vi "Queue Remove.vi"(6 "timeout(ms: -1)":i32=-1, 8 "error in (no error)":errorcluster, 11 "queue name":string) -> (0 "error out":errorcluster, 1 "timeout？":bool, 2 "data":variant, 3 "event":string)   [LabVIEW 2020]
uses:
  Control/Queue Data.ctl
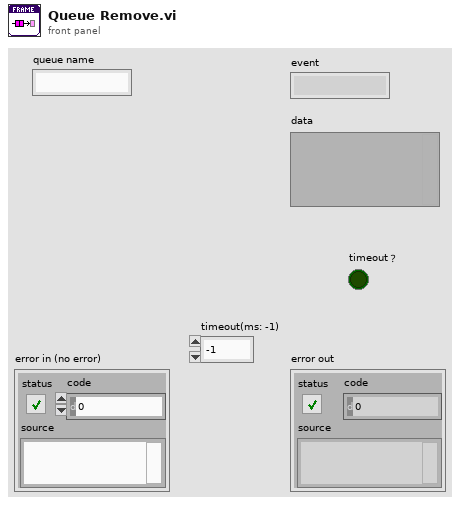
[diagram p1: front panel]
types:
  T1 = typedef "Queue Data.ctl" = cluster{"event":string, "data":variant}
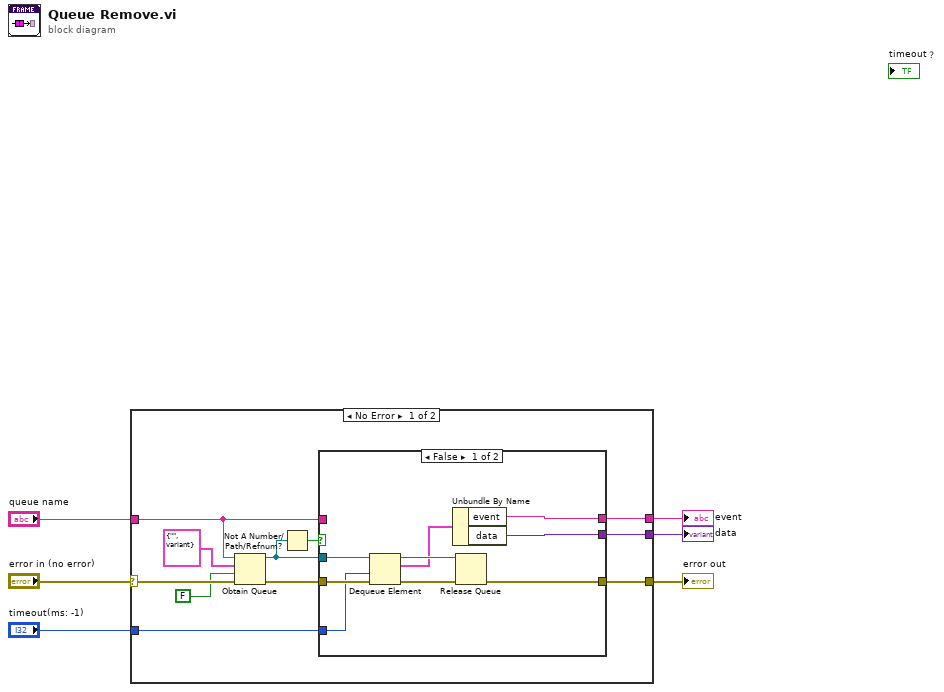
[diagram p0: block diagram]
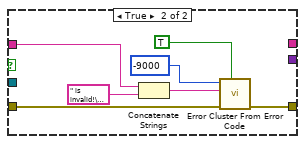
[diagram p2: hidden frame]
diagram:
  n1 = case shown="No Error" "error in (no error)" {
    selector: "error in (no error)" -> [w17 w34]
    tunnel: [w11 w34] -> w5
    tunnel: "queue name" -> [w12 _]
    tunnel: "timeout(ms: -1)" -> [w9 _]
    tunnel: [w8 _] -> w2
    tunnel: [w7 _] -> w1
    frame No Error {
      n2 = Obtain Queue(name (unnamed)=w12, element data type=T1 {"event"="", "data"=variant} ("Cluster"), create if not found? (T)=FALSE, error in (no error)=w17) -> (queue out=w10:refnum<queue>, error out=w14:errorcluster)  [unwired: 1 in, 1 out]
      n3 = Not A Number/Path/Refnum?(number/path/refnum=w10) -> (NaN/Path/Refnum?=w13:bool)
      n4 = case shown="False" w13 {
        tunnel: w14 -> [w26 w29]
        tunnel: w12 -> [_ w28]
        tunnel: [w20 w27] -> w11
        tunnel: w10 -> [w25 _]
        tunnel: w9 -> [w24 _]
        tunnel: [w19 _] -> w7
        tunnel: [w18 _] -> w8
        frame False {
          n5 = Dequeue Element(queue=w25, timeout in ms (-1)=w24, error in (no error)=w26) -> (queue out=w23:refnum<queue>, element=w21:T1, error out=w22:errorcluster)  [unwired: 1 out]
          n6 = Unbundle By Name(w21) -> ("event"=w18:string, "data"=w19:variant)
          n7 = Release Queue(queue=w23, error in (no error)=w22) -> (error out=w20:errorcluster)  [unwired: 1 in, 2 out]
        }
        frame True {
          n8 = Concatenate Strings(w28, " is invalid!\nEnsure the queue has been created!" ("字符串")) -> (w31:string)
          n9 = call <vilib>:"Error Cluster From Error Code.vi"("show call chain? (False)"=TRUE, "error in (no error)"=w29, "error message (\"\")"=w31, "error code (0)"=-9000) -> ("error out"=w27:errorcluster)  [unwired: 5 in]
        }
      }
    }
    frame Error {
    }
  }
  "error out" <- w5
  "event" <- w2
  "data" <- w1
